vi "Otm Cal Acq State.vi"() -> ()   [LabVIEW 2017]
panel:
  out "是否切换时间段？":bool
  out "每时间段开始时间":dbl[](array[numeric])
  out "已循环次数":dbl
  out "当前时间段":i32
  out "是否扫描？":bool
  in  "扫描时间":dbl[](array[numeric])
  in  "持续时间":dbl[](array[numeric])
  in  "运行时间":dbl
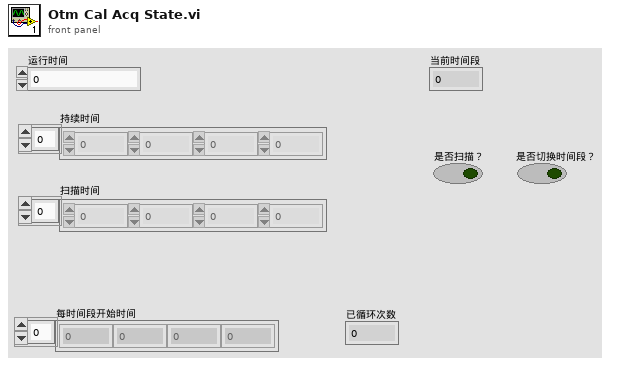
[diagram p1: front panel]
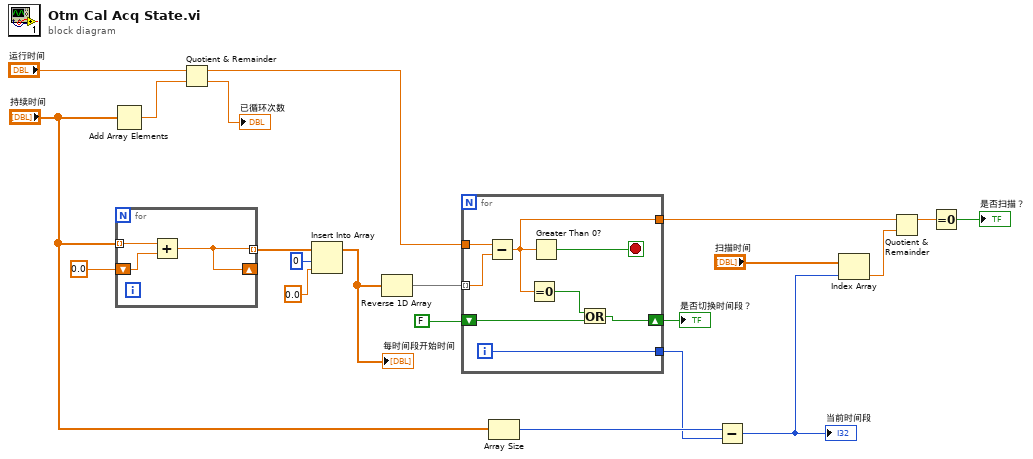
[diagram p0: block diagram]
diagram:
  n1 = Add Array Elements(numeric array="持续时间") -> (sum=w20:dbl)
  n2 = for {
    tunnel: "持续时间" -> [w24] mode=indexing
    shift-right: [w22] -> _
    shift-left: 0.0 -> [w23]
    tunnel: [w22] -> w11 mode=indexing
    n3 = Add(x=w24, y=w23) -> (x+y=w22:dbl)
  }
  n4 = Quotient & Remainder(x="运行时间", y=w20) -> (x-y*floor(x/y)=w17:dbl, floor(x/y)=→"已循环次数":dbl)
  n5 = Insert Into Array(array=w11, index=0, new element=0.0) -> (w10:dbl[])
  "每时间段开始时间" <- w10
  n6 = Reverse 1D Array(array=w10) -> (reversed array=w16:dbl[])
  n7 = for {
    tunnel: w17 -> [w31]
    tunnel: w16 -> [w30] mode=indexing
    tunnel: [w32] -> w14
    shift-right: [w26] -> w7
    shift-left: FALSE -> [w27]
    tunnel: [w25] -> w4
    i -> [w32]
    stop <- w29 stop-if-true
    n8 = Subtract(x=w31, y=w30) -> (x-y=w25:dbl)
    n9 = Equal To 0?(x=w25) -> (x = 0?=w28:bool)
    n10 = Greater Than 0?(x=w25) -> (x > 0?=w29:bool)
    n11 = Or(x=w28, y=w27) -> (x .or. y?=w26:bool)
  }
  "是否切换时间段？" <- w7
  n12 = Array Size(array="持续时间") -> (size(s)=w15:i32)
  n13 = Subtract(x=w15, y=w14) -> (x-y=w5:i32)
  "当前时间段" <- w5
  n14 = Index Array(array="扫描时间", index=w5) -> (element=w3:dbl)
  n15 = Quotient & Remainder(x=w4, y=w3) -> (x-y*floor(x/y)=w2:dbl)  [unwired: 1 out]
  n16 = Equal To 0?(x=w2) -> (x = 0?=→"是否扫描？":bool)
